vi "Setup Check Pressure (SubVI).vi"(5 "Units":u16(ring), 6 "[error source] (\" \")":string, 7 "Labels Array":string[](array[string]), 8 "error in (no error)":errorcluster, 9 "[error source] (\" \") 2":string, 10 "Boolean Array":bool[](array[boolean]), 11 "Channel Array":tag[](array[tag])) -> (0 "error out":errorcluster, 1 "Cluster Out":T1(array[cluster]))   [LabVIEW 2012]
uses:
  <vilib>/Utility/error.llb/DialogType.ctl
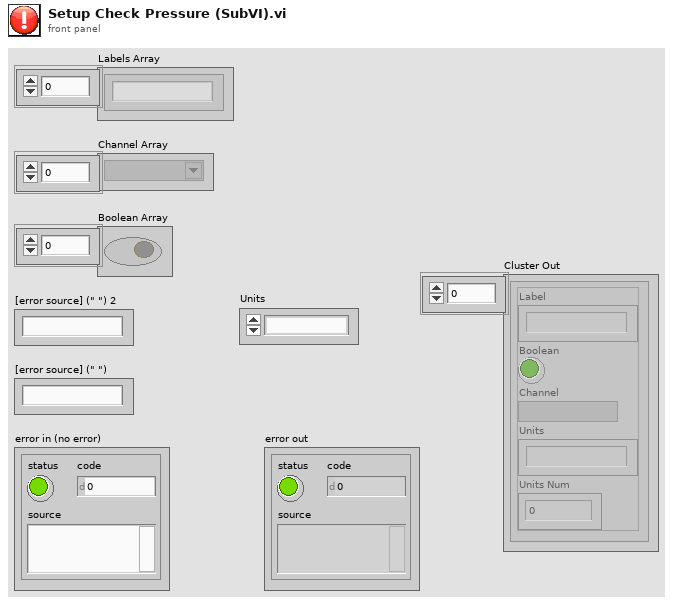
[diagram p1: front panel]
types:
  T1 = cluster{"Label":string, "Boolean":bool, "Channel":tag, "Units":string, "Units Num":i32}[]
  T2 = typedef "DialogType.ctl" = u16
  T3 = cluster{"Label":string, "Boolean":bool, "Channel":tag, "Units":string, "Units Num":i32}
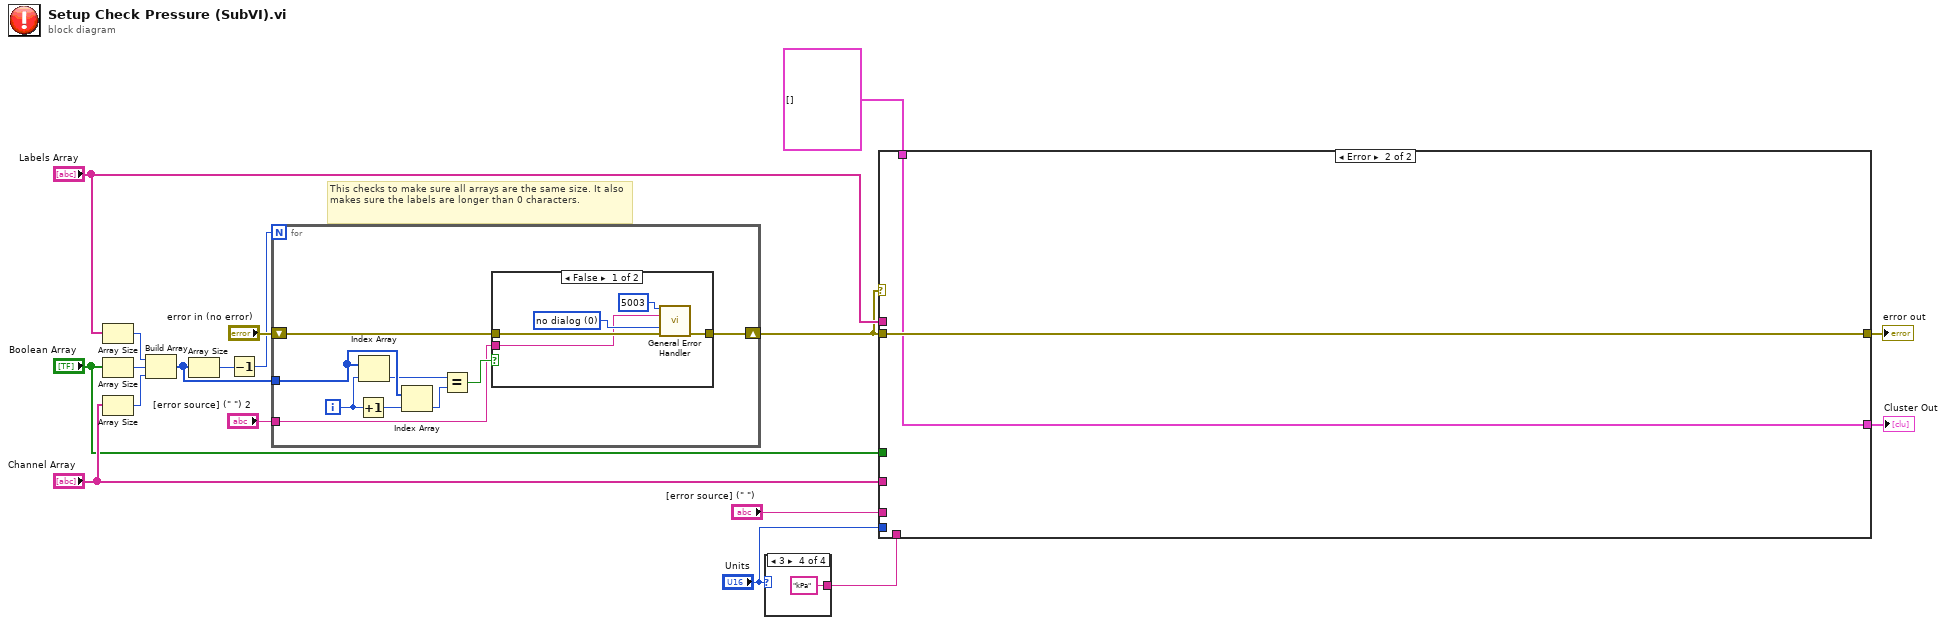
[diagram p0: block diagram]
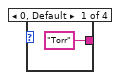
[diagram p2: hidden frame]
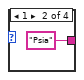
[diagram p3: hidden frame]
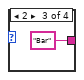
[diagram p4: hidden frame]
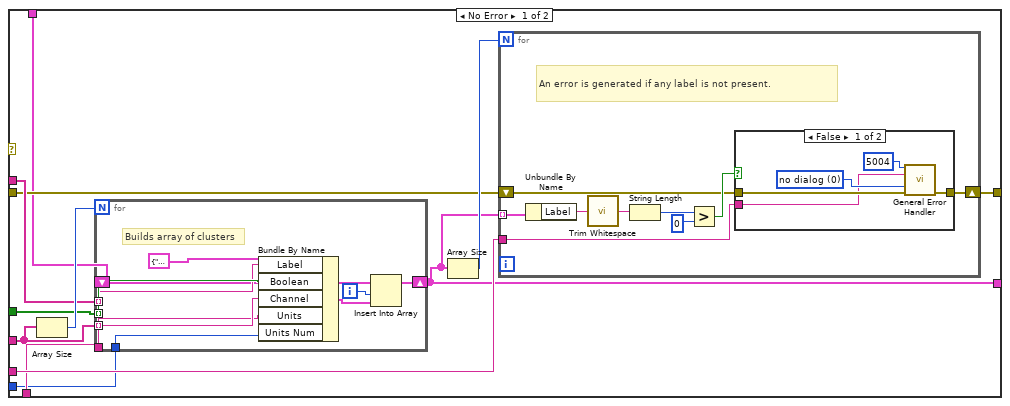
[diagram p5: hidden frame]
diagram:
  # "This checks to make sure all arrays are the same size. It also makes sure the labels are longer than 0 characters."
  n1 = Array Size(array="Labels Array") -> (size(s)=w5:i32)
  n2 = Array Size(array="Boolean Array") -> (size(s)=w6:i32)
  n3 = Array Size(array="Channel Array") -> (size(s)=w7:i32)
  n4 = Build Array(w5, w6, w7) -> (w11:i32[])
  n5 = Array Size(array=w11) -> (size(s)=w8:i32)
  n6 = Decrement(x=w8) -> (x-1=w9:i32)
  n7 = for {
    N: w9 -> [_]
    tunnel: w11 -> [w27]
    tunnel: "[error source] (\" \") 2" -> [w19]
    shift-right: [w20] -> w13
    shift-left: "error in (no error)" -> [w21]
    i -> [w25]
    n8 = Increment(x=w25) -> (x+1=w26:i32)
    n9 = Index Array(array=w27, index=w25) -> (element=w24:i32)
    n10 = Index Array(array=w27, index=w26) -> (element=w23:i32)
    n11 = Equal?(x=w24, y=w23) -> (x = y?=w22:bool)
    n12 = case shown="False" w22 {
      tunnel: w21 -> [w32 w33]
      tunnel: [w31 w33] -> w20
      tunnel: w19 -> [w28 _]
      frame False {
        w30 = T2 0 items=["no dialog", "OK message", "continue or stop message", "OK message + warnings", "continue/stop + warnings"] ("type of dialog (OK msg:1)")
        n13 = call <vilib>:"General Error Handler.vi"("[error code] (0)"=5003, "[error source] (\" \")"=w28, "type of dialog (OK msg:1)"=w30, "error in (no error)"=w32) -> ("error out"=w31:errorcluster)  [unwired: 7 in, 4 out]
      }
      frame True {
      }
    }
  }
  n14 = case shown="3" "Units" {
    tunnel: ["Torr" "Psia" "Bar" "kPa"] -> w4
    frame 0, Default {
    }
    frame 1 {
    }
    frame 2 {
    }
    frame 3 {
    }
  }
  n15 = case shown="Error" w13 {
    tunnel: "Labels Array" -> [w47 _]
    tunnel: "Boolean Array" -> [w46 _]
    tunnel: "Channel Array" -> [w48 _]
    tunnel: [w42 w76] -> w15
    tunnel: w13 -> [w43 w76]
    tunnel: "[error source] (\" \")" -> [w44 _]
    tunnel: w4 -> [w41 _]
    tunnel: "Units" -> [w40 _]
    tunnel: T1 [] -> [w39 w75]
    tunnel: [w38 w75] -> w1
    frame No Error {
      n16 = Array Size(array=w48) -> (size(s)=w49:i32)
      n17 = for {
        N: w49 -> [_]
        tunnel: w46 -> [w73] mode=indexing
        tunnel: w48 -> [w74] mode=indexing
        tunnel: w47 -> [w72] mode=indexing
        tunnel: w41 -> [w70]
        tunnel: w40 -> [w68]
        shift-right: [w66] -> w38
        shift-left: w39 -> [w65]
        i -> [w71]
        # "Builds array of clusters"
        n18 = Bundle By Name(cluster=T3 {"Label"="", "Boolean"=TRUE, "Channel"="", "Units"="", "Units Num"=0}, "Label"=w72, "Boolean"=w73, "Channel"=w74, "Units"=w70, "Units Num"=w68) -> (w67:T3)
        n19 = Insert Into Array(array=w65, index=w71, new element=w67) -> (w66:T1)
      }
      n20 = Array Size(array=w38) -> (size(s)=w45:i32)
      n21 = for {
        N: w45 -> [_]
        shift-right: [w52] -> w42
        shift-left: w43 -> [w53]
        tunnel: w44 -> [w51]
        tunnel: w38 -> [w50] mode=indexing
        # "An error is generated if any label is not present."
        n22 = Unbundle By Name(w50) -> ("Label"=w58:string)
        n23 = call <vilib>:"Trim Whitespace.vi"("string"=w58) -> ("trimmed string"=w57:string)  [unwired: 1 in]
        n24 = String Length(string=w57) -> (length=w56:i32)
        n25 = Greater?(x=w56, y=0) -> (0:w54:bool)
        n26 = case shown="False" w54 {
          tunnel: w53 -> [w61 w64]
          tunnel: [w60 w64] -> w52
          tunnel: w51 -> [w59 _]
          frame False {
            w62 = T2 0 items=["no dialog", "OK message", "continue or stop message", "OK message + warnings", "continue/stop + warnings"] ("type of dialog (OK msg:1)")
            n27 = call <vilib>:"General Error Handler.vi"("[error code] (0)"=5004, "[error source] (\" \")"=w59, "type of dialog (OK msg:1)"=w62, "error in (no error)"=w61) -> ("error out"=w60:errorcluster)  [unwired: 7 in, 4 out]
          }
          frame True {
          }
        }
      }
    }
    frame Error {
    }
  }
  "error out" <- w15
  "Cluster Out" <- w1
